vi "img_read_image (2).vi"(6 "Frame Number":i64=-1, 8 "error in":errorcluster, 9 "Sector size (512)":u32=512, 10 "Image In":T1, 11 "hFile":i64) -> (0 "error out":errorcluster, 1 "lpNumberOfBytesRead":u32, 2 "Image Out":T1, 3 "hFile out":i64)   [LabVIEW 2014]
doc: "This VI reads an image from file using the Win API function ReadFile()."
uses:
  <vilib>/vision/Image Controls.llb/IMAQ Image.ctl
  kernel32.dll
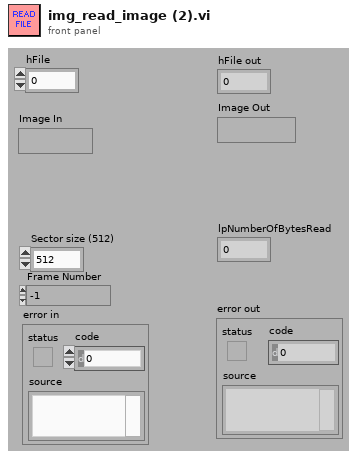
[diagram p1: front panel]
types:
  T1 = typedef "IMAQ Image.ctl" = refnum<image>
  T2 = enum32{"Map Pixel Pointer", "Unmap Pixel Pointer", "Get Pixels Infos"}
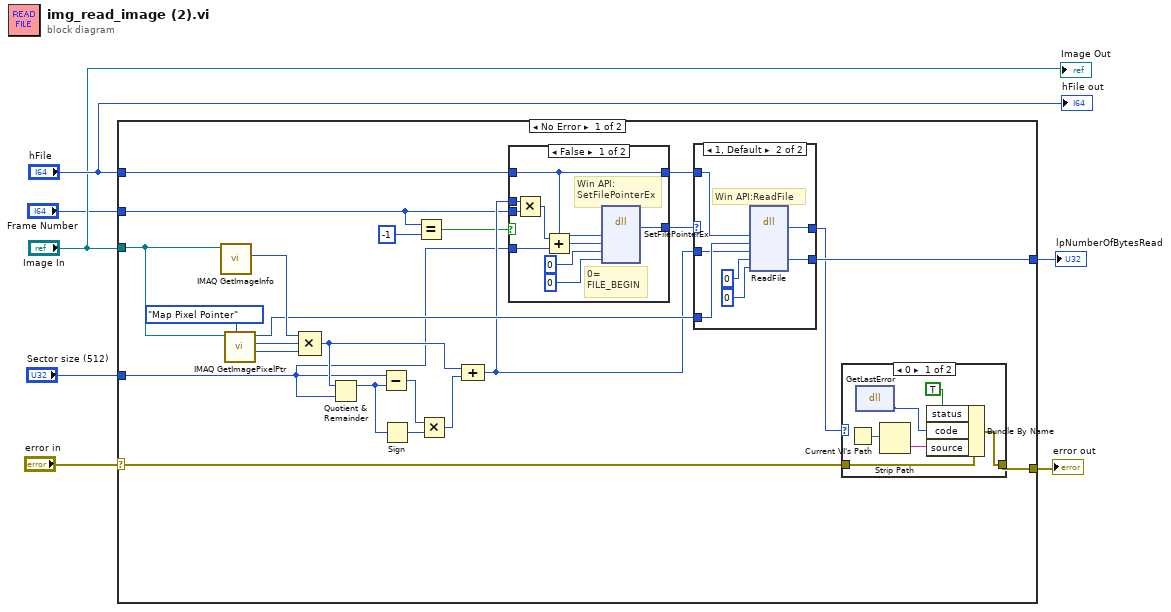
[diagram p0: block diagram]
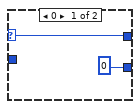
[diagram p2: hidden frame]
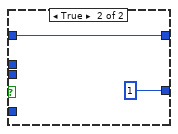
[diagram p3: hidden frame]
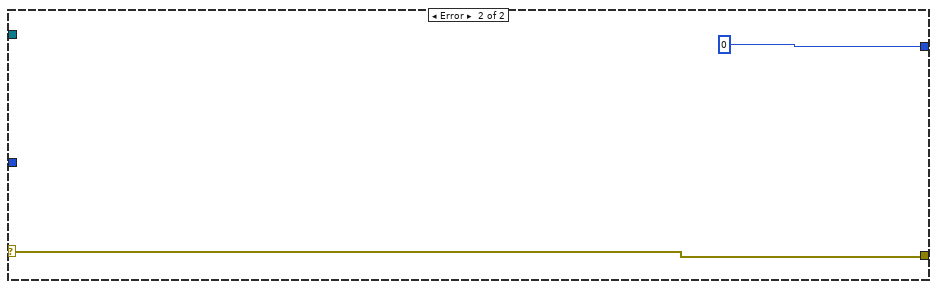
[diagram p5: hidden frame]
diagram:
  n1 = case shown="No Error" "error in" {
    selector: "error in" -> [w12 w59]
    tunnel: "hFile" -> [w16 _]
    tunnel: "Image In" -> [w29 _]
    tunnel: [w24 u32 0 ("lpNumberOfBytesWritten")] -> w5
    tunnel: [w18 w59] -> w3
    tunnel: "Sector size (512)" -> [w9 _]
    tunnel: "Frame Number" -> [w8 _]
    frame No Error {
      n2 = call "IMAQ GetImageInfo"("Image"=w29) -> ("Y Resolution"=w26:i32)  [unwired: 1 in, 9 out]
      n3 = call "IMAQ GetImagePixelPtr"("Function"=T2."Map Pixel Pointer", "Image"=w29) -> ("Pixel Size (Bytes)"=w27:i32, "LineWidth(Pixels)"=w28:i32, "Pixel Pointer out"=w23:u64)  [unwired: 4 in, 3 out]
      n4 = Compound Arithmetic op=MULTIPLY(w26, w28, w27) -> (w25:i32)
      n5 = Quotient & Remainder(x=w25, y=w9) -> (x-y*floor(x/y)=w21:u32)  [unwired: 1 out]
      n6 = Subtract(x=w9, y=w21) -> (x-y=w20:u32)
      n7 = Sign(1:w21) -> (0:w22:u32)
      n8 = Equal?(x=w8, y=i64 -1 ("Frame Number")) -> (x = y?=w10:bool)
      n9 = Multiply(x=w20, y=w22) -> (x*y=w19:u32)
      n10 = Compound Arithmetic op=ADD(w25, w19) -> (w15:u32)
      n11 = case shown="False" w10 {
        tunnel: w8 -> [w48 _]
        tunnel: w16 -> [w43 w50]
        tunnel: w15 -> [w47 _]
        tunnel: [w43 w50] -> w14
        tunnel: [w42 1 ("error")] -> w13
        tunnel: w9 -> [w40 _]
        frame False {
          # "Win API:\nSetFilePointerEx"
          # "0=\nFILE_BEGIN"
          n12 = Multiply(x=w47, y=w48) -> (x*y=w46:i64)
          n13 = Add(x=w46, y=w40) -> (x+y=w41:i64)
          n14 = dll-call lib="kernel32.dll" fn="SetFilePointerEx"("hFile"=w43, "lDistanceToMove"=w41, "lpNewFilePointer"=i64 0, "dwMoveMethod"=u32 0) -> ("error"=w42:i32)  [unwired: 5 in, 4 out]
        }
        frame True {
        }
      }
      n15 = case shown="1, Default" w13 {
        selector: w13 -> [w32 _]
        tunnel: [u32 0 ("lpNumberOfBytesRead") w39] -> w24
        tunnel: w23 -> [_ w37]
        tunnel: [w32 w35] -> w17
        tunnel: w15 -> [_ w34]
        tunnel: w14 -> [_ w33]
        frame 0 {
        }
        frame 1, Default {
          # "Win API:ReadFile"
          n16 = dll-call lib="kernel32.dll" fn="ReadFile"("hFile"=w33, "lpBuffer"=w37, "nNumberOfBytesToRead"=w34, "lpNumberOfBytesRead"=u32 0 ("lpOverlapped"), "lpOverlapped"=u32 0) -> ("error"=w35:i32, "lpNumberOfBytesRead"=w39:u32)  [unwired: 6 in, 3 out]
        }
      }
      n17 = case shown="0" w17 {
        tunnel: w12 -> [w56 w57]
        tunnel: [w55 w57] -> w18
        frame 0 {
          n18 = Current VI's Path() -> (path=w53:path)
          n19 = dll-call lib="kernel32.dll" fn="GetLastError"() -> ("error"=w51:u32)  [unwired: 3 in, 2 out]
          n20 = Strip Path(path=w53) -> (name=w52:string)  [unwired: 1 out]
          n21 = Bundle By Name(cluster=w56, "status"=TRUE, "code"=w51, "source"=w52) -> (w55:errorcluster)
        }
        frame 1, Default {
        }
      }
    }
    frame Error {
    }
  }
  "lpNumberOfBytesRead" <- w5
  "error out" <- w3
  "Image Out" <- "Image In"
  "hFile out" <- "hFile"
